vi "Afterpulsing calculation.vi"(10 "Histogram with 128 ns bin":i64[](array[numeric]), 11 "Total counts":i64) -> (3 "Afterpulsing probability (%)":dbl)   [LabVIEW 2012]
uses:
  <vilib>/Analysis/6fits.llb/Curve Fitting Criteria.ctl
  <vilib>/Analysis/NI_AALPro.lvlib
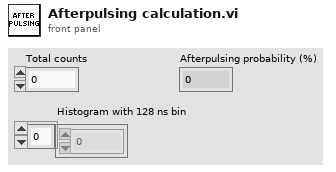
[diagram p1: front panel]
types:
  T1 = cluster{"amp min":dbl, "amp max":dbl, "damping min":dbl, "damping max":dbl, "offset min":dbl, "offset max":dbl}
  T2 = typedef "NI_AALPro.lvlib/Curve Fitting Criteria.ctl" = u16
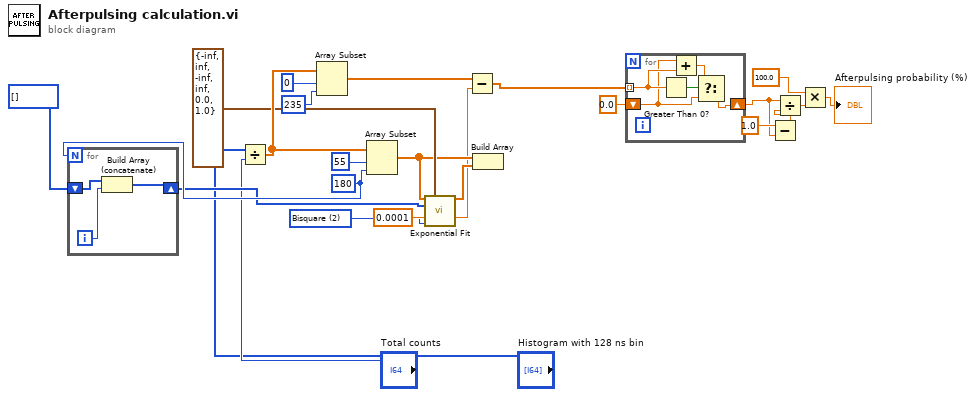
[diagram p0: block diagram]
diagram:
  w20 = T2 2 items=["Least Square", "Least Absolute Residual", "Bisquare"] ("method")
  w19 = 180 ("length")
  n1 = for {
    N: w19 -> [_]
    shift-right: [w27] -> w5
    shift-left: i32[] [] -> [w25]
    i -> [w26]
    n2 = Build Array (concatenate)(w25, w26) -> (w27:i32[])
  }
  n3 = Divide(x="Histogram with 128 ns bin", y="Total counts") -> (x/y=w23:dbl[])
  n4 = Array Subset(array=w23, index=0, length=235) -> (w8:dbl[])
  n5 = Array Subset(array=w23, index=55, length=w19) -> (w17:dbl[])
  n6 = call <vilib>:"Exponential Fit.vi"("Y"=w17, "X"=w5, "tolerance"=0.0001, "method"=w20, "parameter bounds"=T1 {"amp min"=-inf, "amp max"=inf, "damping min"=-inf, "damping max"=inf, "offset min"=0.0, "offset max"=1.0}) -> ("Best Exponential Fit"=w18:dbl[], "offset"=w9:dbl)  [unwired: 5 in, 4 out]
  n7 = Subtract(x=w8, y=w9) -> (x-y=w24:dbl[])
  n8 = Build Array(w17, w18) -> ()  [unwired: 1 out]
  n9 = for {
    tunnel: w24 -> [w30] mode=indexing
    shift-right: [w31] -> w11
    shift-left: 0.0 -> [w29]
    n10 = Greater Than 0?(x=w30) -> (x > 0?=w32:bool)
    n11 = Add(x=w29, y=w30) -> (x+y=w28:dbl)
    n12 = Select(t=w28, s=w32, f=w29) -> (s? t:f=w31:dbl)
  }
  n13 = Subtract(x=1.0, y=w11) -> (x-y=w13:dbl)
  n14 = Divide(x=w11, y=w13) -> (x/y=w14:dbl)
  n15 = Multiply(x=100.0, y=w14) -> (x*y=→"Afterpulsing probability (%)":dbl)
